vi "Change_RunNumber.vi"(6 "Valid Run Number":i32, 7 "Changing the run number?":bool, 8 "error in (no error)":errorcluster, 9 "Array":dbl[](array[numeric]), 10 "String in":string, 11 "path in":path) -> (0 "error out":errorcluster, 3 "String out":string)   [LabVIEW 2019]
panel:
  out "Proposed Run Number":i32
  in  "Apply Run Number?":bool
  in  "New Run Number":i32
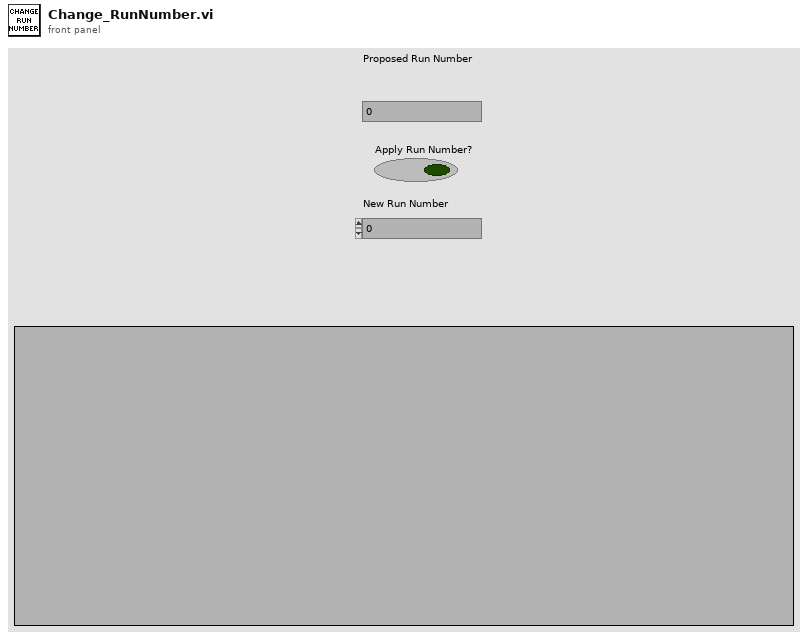
[diagram p1: front panel]
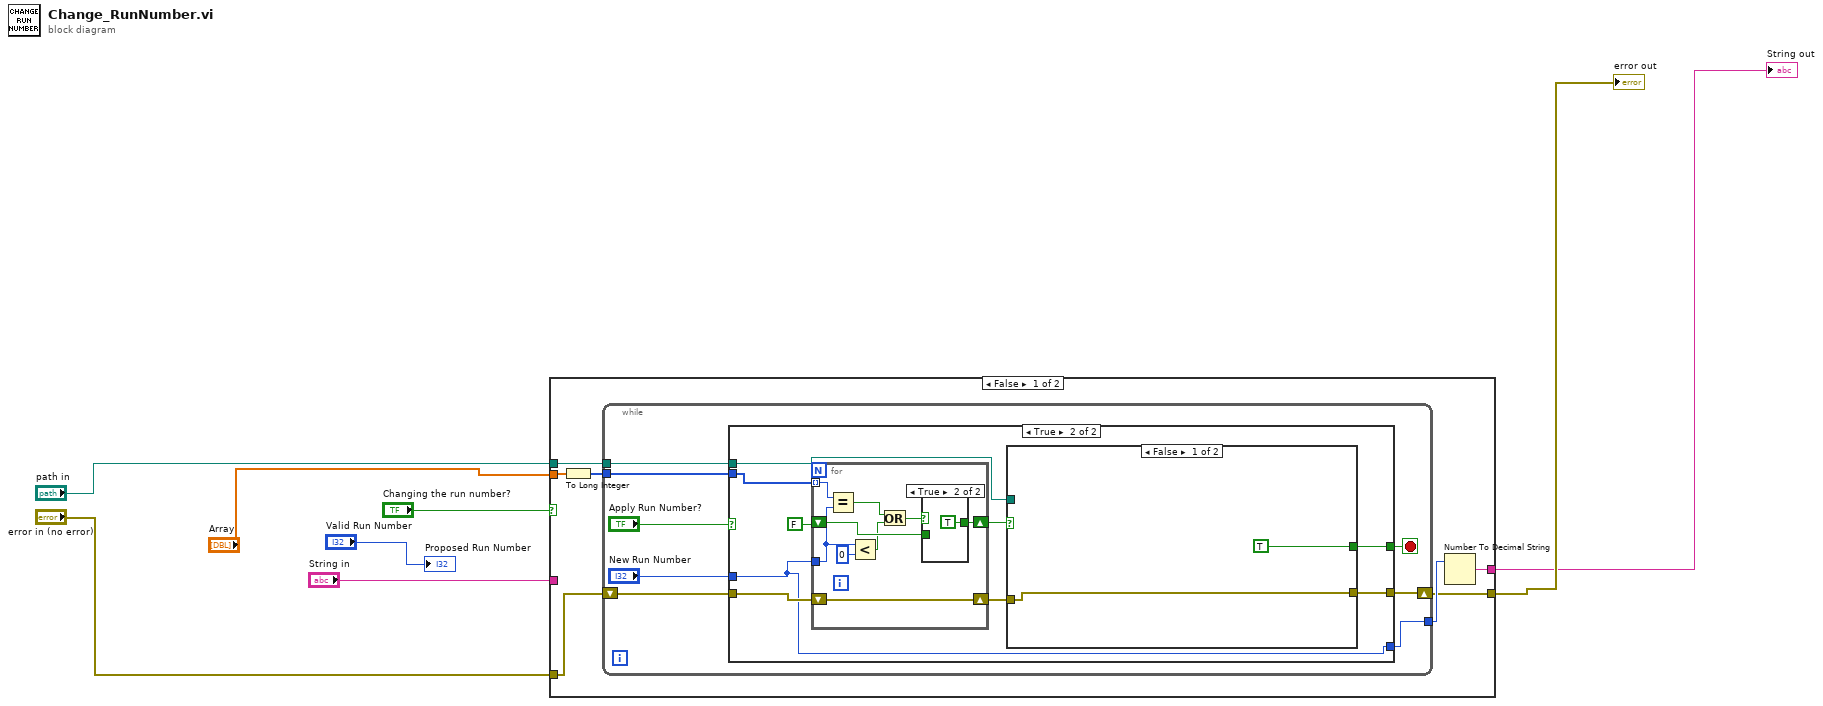
[diagram p0: block diagram]
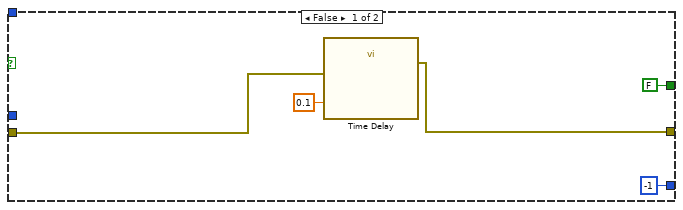
[diagram p2: hidden frame]
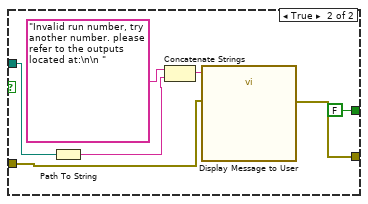
[diagram p3: hidden frame]
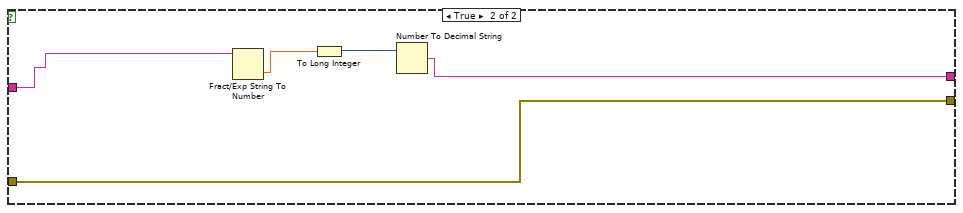
[diagram p5: hidden frame]
diagram:
  n1 = case shown="False" "Changing the run number?" {
    tunnel: "Array" -> [w15 _]
    tunnel: "path in" -> [w13 _]
    tunnel: "error in (no error)" -> [w12 w62]
    tunnel: [w10 w62] -> w8
    tunnel: [w9 w58] -> w7
    tunnel: "String in" -> [_ w61]
    frame False {
      n2 = To Long Integer(number=w15) -> (32bit integer=w14:i32[])
      n3 = while {
        tunnel: w14 -> [w22]
        tunnel: w13 -> [w20]
        shift-right: [w18] -> w10
        shift-left: w12 -> [w19]
        tunnel: [w16] -> w11
        stop <- w17 stop-if-true
        n4 = case shown="True" "Apply Run Number?" {
          tunnel: w22 -> [_ w37]
          tunnel: "New Run Number" -> [_ w29]
          tunnel: w20 -> [_ w34]
          tunnel: w19 -> [w27 w32]
          tunnel: [w26 w31] -> w18
          tunnel: [FALSE w30] -> w17
          tunnel: [-1 ("Enter Number") w29] -> w16
          frame False {
            n5 = call "Time Delay"("error in (no error)"=w27, "Delay Time (s)"=0.1) -> ("error out"=w26:errorcluster)  [unwired: 9 in]
          }
          frame True {
            n6 = for {
              tunnel: w37 -> [w55] mode=indexing
              tunnel: w29 -> [w51]
              shift-right: [w53] -> w35
              shift-left: FALSE -> [w54]
              shift-right: [w52] -> w33
              shift-left: w32 -> [w52]
              n7 = Equal?(x=w55, y=w51) -> (x = y?=w48:bool)
              n8 = Less?(x=w51, y=0) -> (x < y?=w49:bool)
              n9 = Or(x=w48, y=w49) -> (x .or. y?=w47:bool)
              n10 = case shown="True" w47 {
                tunnel: w54 -> [w56 _]
                tunnel: [w56 TRUE] -> w53
                frame False {
                }
                frame True {
                }
              }
            }
            n11 = case shown="False" w35 {
              tunnel: w34 -> [_ w44]
              tunnel: w33 -> [w39 w42]
              tunnel: [w39 w41] -> w31
              tunnel: [TRUE FALSE] -> w30
              frame False {
              }
              frame True {
                n12 = Path To String(path=w44) -> (string=w43:string)
                n13 = Concatenate Strings("Invalid run number, try another number. please refer to the outputs located at:\n\n ", w43) -> (w45:string)
                n14 = call "Display Message to User"("error in (no error)"=w42, "Message"=w45) -> ("error out"=w41:errorcluster)  [unwired: 8 in, 1 out]
              }
            }
          }
        }
      }
      n15 = Number To Decimal String(number=w11) -> (decimal integer string=w9:string)  [unwired: 1 in]
    }
    frame True {
      n16 = Fract/Exp String To Number(string=w61) -> (number=w59:dbl)  [unwired: 3 in, 1 out]
      n17 = To Long Integer(number=w59) -> (32bit integer=w60:i32)
      n18 = Number To Decimal String(number=w60) -> (decimal integer string=w58:string)  [unwired: 1 in]
    }
  }
  "error out" <- w8
  "String out" <- w7
  "Proposed Run Number" <- "Valid Run Number"
